vi "SMC_Getvel.vi"(8 "error in (no error)":errorcluster) -> (0 "error out":errorcluster, 2 "Velocity":dbl format="%.2f")   [LabVIEW 2015]
uses:
  SMC_SubVIs.llb/SMC_ManagerMode.ctl
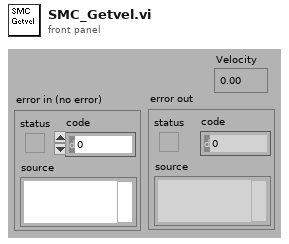
[diagram p1: front panel]
types:
  T1 = typedef "SMC_ManagerMode.ctl" = enum16{"Init", "Get", "SetPosition", "SetStatus", "SetMoving", "SetControllerNr"}
  T2 = typedef "SMC Paras.ctl" = cluster{"VENUS Language":T3, "Number of Axis":u8, "Controller Nr":u8, "Simulation":bool}
  T3 = typedef "VENUSNr.ctl" = enum16{"VENUS 2", "VENUS 1"}
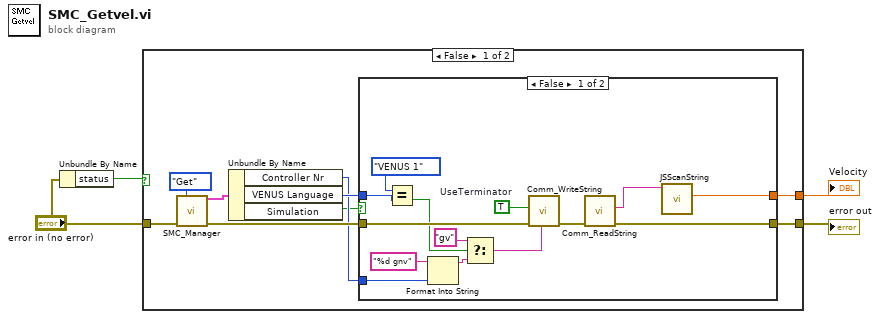
[diagram p0: block diagram]
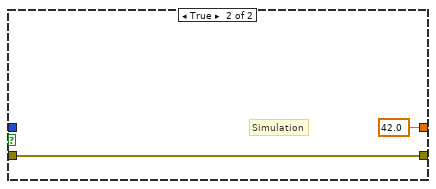
[diagram p2: hidden frame]
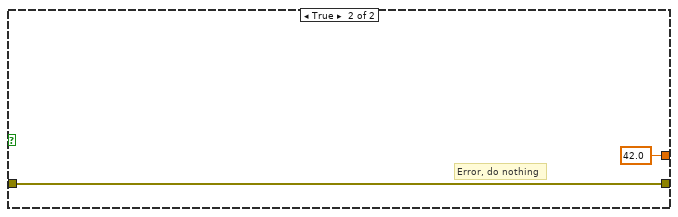
[diagram p3: hidden frame]
diagram:
  n1 = Unbundle By Name("error in (no error)") -> ("status"=w4:bool)
  n2 = case shown="False" w4 {
    tunnel: "error in (no error)" -> [w12 w31]
    tunnel: [w10 w31] -> w2
    tunnel: [w9 42.0 ("result")] -> w1
    frame False {
      n3 = call "SMC_Manager.vi"("Mode"=SMC_ManagerMode."Get", "error in (no error)"=w12) -> ("SMC Parameter Out"=w8:T2, "error out"=w11:errorcluster)  [unwired: 9 in, 3 out]
      n4 = Unbundle By Name(w8) -> ("Controller Nr"=w6:u8, "VENUS Language"=w7:T3, "Simulation"=w5:bool)
      n5 = case shown="False" w5 {
        tunnel: w11 -> [w27 w29]
        tunnel: [w25 w29] -> w10
        tunnel: w7 -> [w23 _]
        tunnel: w6 -> [w18 _]
        tunnel: [w15 42.0 ("result")] -> w9
        frame False {
          w14 = TRUE  # UseTerminator
          n6 = Equal?(x=enum16{"VENUS 2", "VENUS 1"}."VENUS 1", y=w23) -> (x = y?=w21:bool)
          n7 = Format Into String(format string="%d gnv" ("Format String"), w18) -> (resulting string=w17:string)  [unwired: 2 in, 1 out]
          n8 = Select(t="gv" ("Substring"), s=w21, f=w17) -> (s? t:f=w19:string)
          n9 = call "Comm_WriteString.vi"("string to write"=w19, "error in (no error)"=w27, "UseTerminator"=w14) -> ("error out"=w26:errorcluster)  [unwired: 8 in]
          n10 = call "Comm_ReadString.vi"("error in (no error)"=w26) -> ("error out"=w25:errorcluster, "Answer"=w16:string)  [unwired: 9 in]
          n11 = call "JSScanString.vi"("String"=w16) -> ("result"=w15:dbl)  [unwired: 9 in, 1 out]
        }
        frame True {
          # "Simulation"
        }
      }
    }
    frame True {
      # "Error, do nothing"
    }
  }
  "error out" <- w2
  "Velocity" <- w1
